vi "Start.vi"(8 "error in":errorcluster, 11 "Rx Execution Unit Implementation in":refnum<class "Rx Execution Unit.lvclass">) -> (0 "error out":errorcluster, 3 "Rx Execution Unit Implementation out":refnum<class "Rx Execution Unit.lvclass">)   [LabVIEW 2020, in "afdx_custom_device Engine.lvlib" / "Implementation.lvlib" / "Rx Execution Unit.lvclass"]
uses:
  Rx Execution Unit.lvclass
  AIM LabVIEW src/src/AIM664LV.lvlib
  afdx_custom_device Engine.lvlib
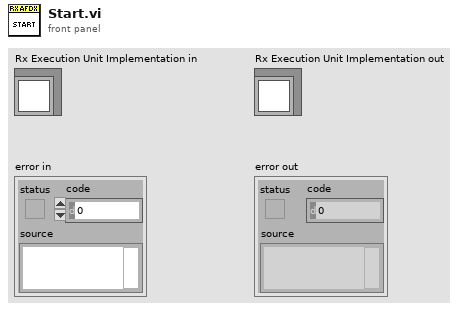
[diagram p1: front panel]
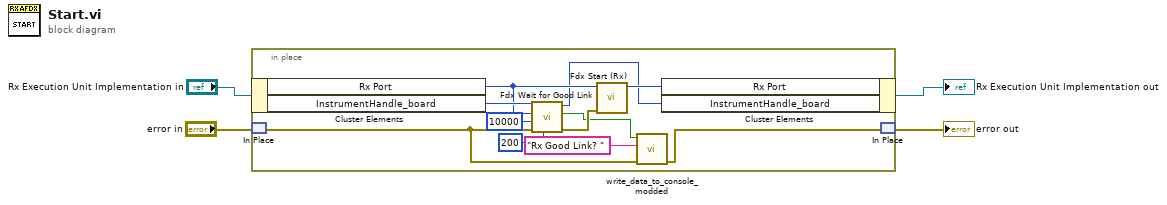
[diagram p0: block diagram]
diagram:
  n1 = in-place {
    n2 = in-place-cluster #1("Rx Execution Unit Implementation in") -> ("Rx Port"=w12:u32, "InstrumentHandle_board"=w13:u32)
    n3 = in-place-match #2("error in") -> (w8:errorcluster)
    n4 = call "Fdx Wait for Good Link.vi"("retry period (ms)"=u32 200, "error in"=w8, "timeout (ms)"=u32 10000, "port id"=w12, "InstrumentHandle_board in"=w13) -> ("error out"=w14:errorcluster, "good link"=w6:bool, "InstrumentHandle_board out"=w11:u32)  [unwired: 3 in, 1 out]
    n5 = call "Fdx Start (Rx).vi"("error in"=w14, "InstrumentHandle_port in"=w12) -> ("InstrumentHandle_port out"=w15:u32)  [unwired: 8 in, 1 out]
    n6 = call "write_data_to_console_modded.vi"("error in"=w8, "Tag"="Rx Good Link? ", "Data"=w6) -> ("error out"=w7:errorcluster)  [unwired: 8 in]
    n7 = in-place-cluster #1("Rx Port"=w15, "InstrumentHandle_board"=w11) -> (→"Rx Execution Unit Implementation out":refnum<class "Rx Execution Unit.lvclass">)
    n8 = in-place-match #2(w7) -> (→"error out":errorcluster)
  }
